vi "MNK_FP_to_DSC.vi"(0 "str":string[](array[string]), 1 "str var":refnum<k21>[](array[refnum])=["ni.var.psp://housesoftheholy/MNK_18T/MNK_FP_STATE"], 2 "dbl":dbl[](array[numeric]), 3 "dbl var":refnum<k21>[](array[refnum])=["ni.var.psp://housesoftheholy/MNK_18T/MNK_FP_P1", "ni.var.psp://housesoftheholy/MNK_18T/MNK_FP_P2", "ni.var.psp://housesoftheholy/MNK_18T/MNK_FP_P3", "ni.var.psp://housesoftheholy/MNK_18T/MNK_FP_P4", "ni.var.psp://housesoftheholy/MNK_18T/MNK_FP_P5", "ni.var.psp://housesoftheholy/MNK_18T/MNK_FP_P6", "ni.var.psp://housesoftheholy/MNK_18T/MNK_FP_P7", "ni.var.psp://housesoftheholy/MNK_18T/MNK_FP_Flow", "ni.var.psp://housesoftheholy/MNK_18T/MNK_FP_MG0", "ni.var.psp://housesoftheholy/MNK_18T/MNK_FP_MG1", "ni.var.psp://housesoftheholy/MNK_18T/MNK_FP_MG2", "ni.var.psp://housesoftheholy/MNK_18T/MNK_FP_MG3", "ni.var.psp://housesoftheholy/MNK_18T/MNK_FP_MG4", "ni.var.psp://housesoftheholy/MNK_18T/MNK_FP_MG5", "ni.var.psp://housesoftheholy/MNK_18T/MNK_FP_state0", "ni.var.psp://housesoftheholy/MNK_18T/MNK_FP_state1", "ni.var.psp://housesoftheholy/MNK_18T/MNK_FP_state2"]) -> ()   [LabVIEW 2013]
panel:
  # "MNK FP to DSC"
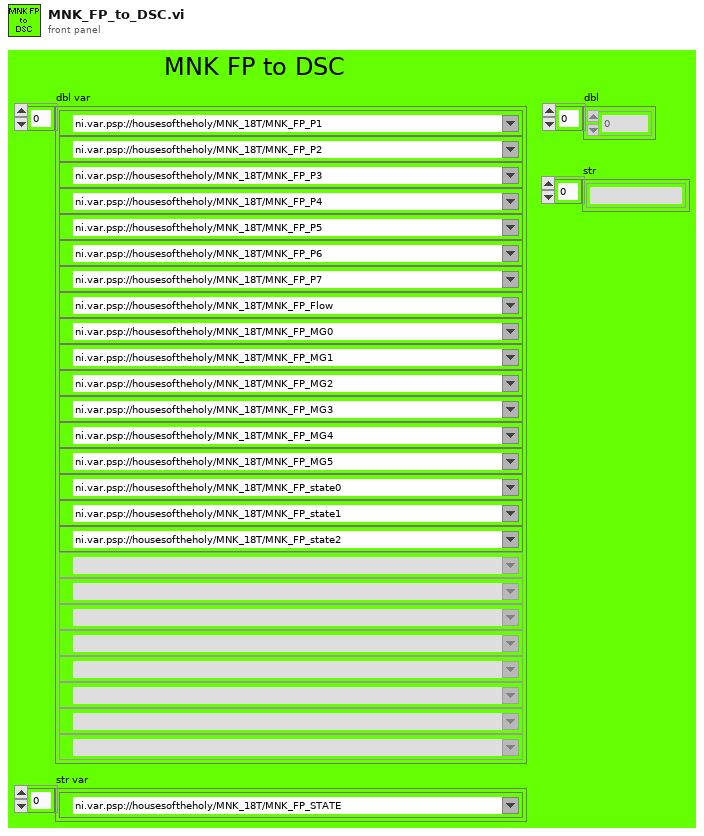
[diagram p1: front panel]
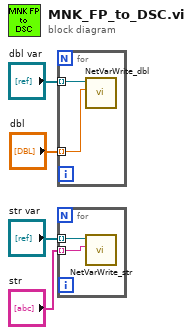
[diagram p0: block diagram]
diagram:
  n1 = for {
    tunnel: "dbl var" -> [w6] mode=indexing
    tunnel: "dbl" -> [w5] mode=indexing
    n2 = call "NetVarWrite_dbl.vi"("Numeric"=w5, "Refnum in"=w6) -> ()  [unwired: 10 in]
  }
  n3 = for {
    tunnel: "str var" -> [w8] mode=indexing
    tunnel: "str" -> [w7] mode=indexing
    n4 = call "NetVarWrite_str.vi"("String"=w7, "Refnum in"=w8) -> ()  [unwired: 10 in]
  }
